vi "PRNG Cipher Stream in LabVIEW.vi"() -> ()   [LabVIEW 2016]
uses:
  <extravilib>/ChannelInstances/One Element Stream-bool/Read With Abort.vi
  <extravilib>/ChannelInstances/One Element Stream-bool/Write With Abort.vi
  <extravilib>/ChannelInstances/One Element Stream-bool/Instantiate.vi
  <extravilib>/ChannelInstances/One Element Stream-bool/EndpointRead.vi
  <extravilib>/ChannelInstances/One Element Stream-bool/Endpoint.vi
  <vilib>/Analysis/NI_AALBase.lvlib
  <extravilib>/ChannelInstances/One Element Stream-bool.lvlib
panel:
  out "Chart 2":dbl(graph)
  in  "seed":i32=-1
  in  "stop":bool
  out "Chart":dbl(graph)
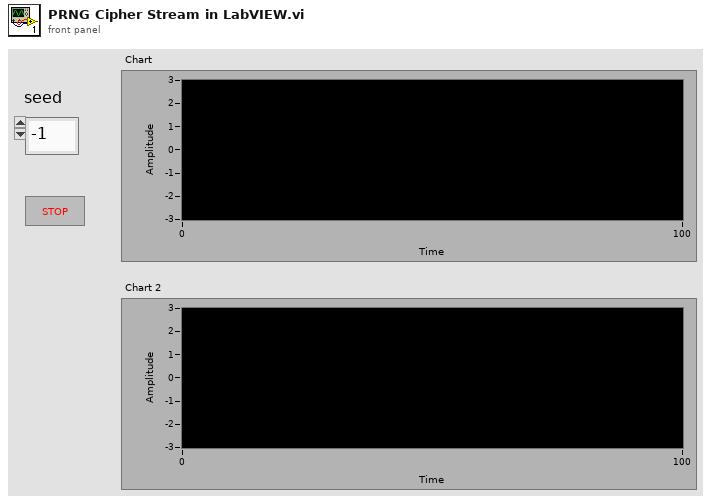
[diagram p1: front panel]
types:
  T1 = typedef "One Element Stream-bool.lvlib/)Channel.ctl" = refnum<queue>
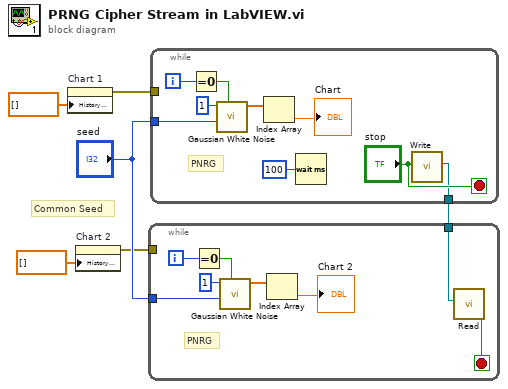
[diagram p0: block diagram]
diagram:
  # "Common Seed"
  n1 = property on="Chart 1" class="WFChart (strict)"("History Data"=dbl[] []) -> (error out=w4:errorcluster)  [unwired: 2 in, 1 out]
  n2 = property on="Chart 2" class="WFChart (strict)"("History Data"=dbl[] []) -> (error out=w1:errorcluster)  [unwired: 2 in, 1 out]
  n3 = while {
    tunnel: "seed" -> [w8]
    tunnel: [w7] -> w5
    tunnel: w4 -> [_]
    i -> [w12]
    stop <- "stop" stop-if-true
    # "PNRG"
    n4 = Equal To 0?(x=w12) -> (x = 0?=w11:bool)
    n5 = call <vilib>:"Gaussian White Noise.vi"("initialize?"=w11, "seed"=w8, "samples"=1) -> ("Gaussian noise pattern"=w14:dbl[])  [unwired: 7 in, 1 out]
    n6 = Index Array(array=w14) -> (element=→"Chart":dbl)  [unwired: 1 in]
    n7 = Wait (ms)(milliseconds to wait=u32 100) -> ()  [unwired: 1 out]
    n8 = call <extravilib>:"Write.vi"("element"="stop") -> ("channel"=w7:T1)  [unwired: 9 in, 1 out]
  }
  n9 = while {
    tunnel: "seed" -> [w18]
    tunnel: w5 -> [w17]
    tunnel: w1 -> [_]
    i -> [w20]
    stop <- w16 stop-if-true
    # "PNRG"
    n10 = Equal To 0?(x=w20) -> (x = 0?=w19:bool)
    n11 = call <vilib>:"Gaussian White Noise.vi"("initialize?"=w19, "seed"=w18, "samples"=1) -> ("Gaussian noise pattern"=w22:dbl[])  [unwired: 7 in, 1 out]
    n12 = Index Array(array=w22) -> (element=→"Chart 2":dbl)  [unwired: 1 in]
    n13 = call <extravilib>:"Read.vi"("channel"=w17) -> ("element"=w16:bool)  [unwired: 7 in, 3 out]
  }
